vi "Initialize.vi"(6 "optional":variant, 8 "error in (no error)":errorcluster, 11 "Node data":refnum<class "Node.lvclass">) -> (0 "error out":errorcluster, 3 "Node out":refnum<data-value>)   [LabVIEW 2009, in "Node.lvclass"]
uses:
  Node.lvclass
  DataObj/DataObj.lvclass
  Node.lvclass/Node.ctl
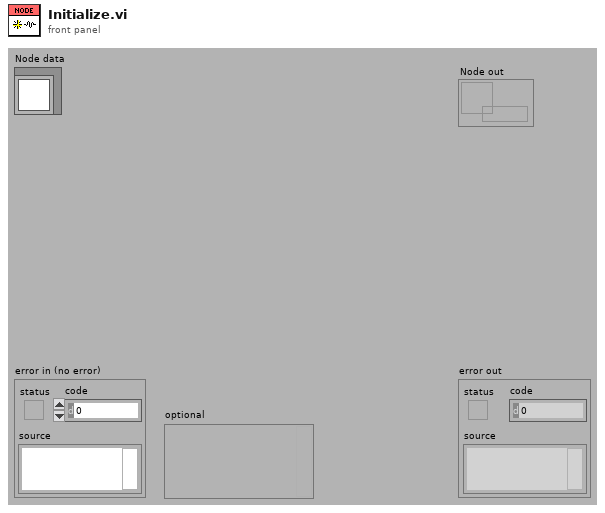
[diagram p1: front panel]
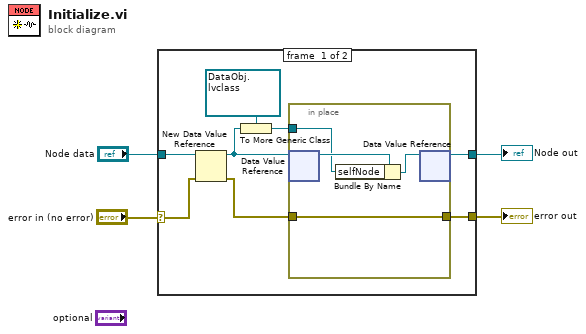
[diagram p0: block diagram]
diagram:
  n1 = case shown="No Error" "error in (no error)" {
    selector: "error in (no error)" -> [w11 w17]
    tunnel: "Node data" -> [w8 _]
    tunnel: [w10 w17] -> w1
    tunnel: [w9 _] -> w2
    frame #0 {
      n2 = New Data Value Reference(data value=w8, error in=w11) -> (data value reference=w6:refnum<data-value>, error out=w12:errorcluster)
      n3 = To More Generic Class(target class=refnum<data-value> refnum ("ID"), reference=w6) -> (generic class reference=w7:refnum<data-value>)
      n4 = in-place {
        in-place-border: w12 -> [w14]
        in-place-border: w7 -> [w13]
        in-place-border: [w14] -> w10
        n5 = in-place-dvr #1(w6) -> (w16:refnum<class "Node.lvclass">)  [unwired: 1 out]
        n6 = Bundle By Name(cluster=w16, "selfNode"=w13) -> (w15:refnum<class "Node.lvclass">)
        n7 = in-place-dvr #1(w15) -> (w9:refnum<data-value>)  [unwired: 1 out]
      }
    }
    frame #1 {
    }
  }
  "error out" <- w1
  "Node out" <- w2
